vi "Read Write_Loop.vi"() -> ()   [LabVIEW 2020, in "NTV Read Write.lvlib"]
uses:
  NTV Read Write.lvlib
  Shared Code/TypeDefs/Dial_Compase heading unit circle CCW positive.ctl
  Shared Code/TypeDefs/Cluster_CMD_Direction Data.ctl
  Shared Code/TypeDefs/Cluster_Module Velocity-Direction-Rotations.ctl
  Shared Code/TypeDefs/Level_Velocity plus-minus 1.ctl
  Shared Code/TypeDefs/ENUM RB_Drive Mode IND.ctl
  Shared Code/TypeDefs/Cluster_Shooter Speed Data.ctl
  Shared Code/TypeDefs/ENUM RB_Feeder State.ctl
  Shared Code/TypeDefs/ENUM_Tube Wheel Positions.ctl
  ENUM_SEN_State.ctl
  ENUM_SEN_Action.ctl
  RoboRIO Utilities/Global_STOP.vi
  PigeonIMU/Global_SEN_Data Out.vi
  SwerveDrive/Global_CMD_ACT_Data In.vi
  Shooter/Global_CMD_ACT_Data In.vi
  Shooter/Global_ACT_Data Out.vi
  Feeder/Global_ACT_Data Out.vi
  Tube Wheel/Global_ACT_Data Out.vi
  Global_SEN_Data Out.vi
  PigeonIMU/PigeonIMU_SEN_ts.lvlib
  SwerveDrive/SwerveDrive_ACT_ts.lvlib
  Shooter/Shooter_ACT.lvlib
  Feeder/Feeder_ACT.lvlib
  Tube Wheel/Tube Wheel_ACT.lvlib
panel:
  out "Current Position":T1
  out "Feeder State":T2
  out "output cluster":T3
  out "Drive Mode":T4
  out "Run Stop":bool
  out "Direction":T5 {"Rotate(Yaw) CCW 1 CW -1" scale=1.0..-1.0; "Traverse"."Angle" scale format="%.3f"; "Traverse"."Velocity" scale=-1.0..1.0 scale format="%.1f"}
  out "Yaw":T8 scale format="%.3f"
  out "Cycle Time (S)":dbl format="%.3g"
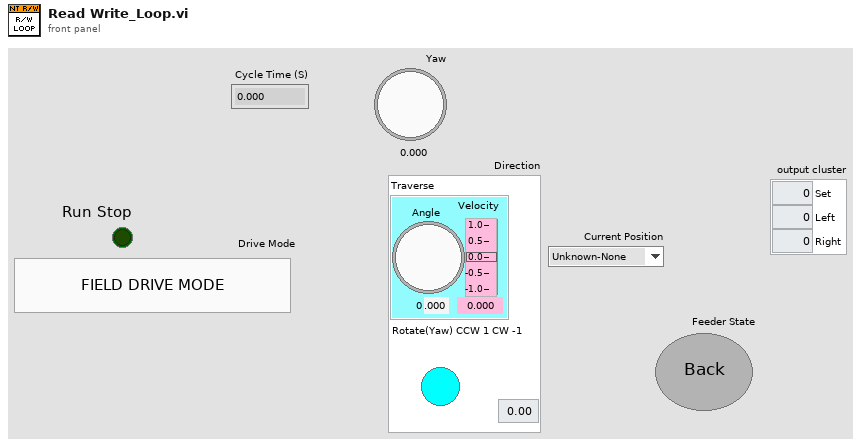
[diagram p1: front panel]
types:
  T1 = typedef "ENUM_Tube Wheel Positions.ctl" = enum16{"Unknown-None", "Tube Red A", "Tube Black B", "Tube Red C", "Tube Black D", "Tube Red E", "Tube Black F", "Load A-B", "Load B-C", "Load C-D", "Load D-E", "Load E-F", "Load F-A"}
  T2 = typedef "ENUM RB_Feeder State.ctl" = enum32{"Back", "Reversing", "Shooting"}
  T3 = typedef "Cluster_Shooter Speed Data.ctl" = cluster{"Set":dbl, "Left":dbl, "Right":dbl}
  T4 = typedef "ENUM RB_Drive Mode IND.ctl" = enum32{"Field Drive Mode", "Robot Drive Mode", "Turrent Drive Mode"}
  T5 = typedef "Cluster_CMD_Direction Data.ctl" = cluster{"Traverse":T6, "Rotate(Yaw) CCW 1 CW -1":dbl}
  T6 = typedef "Cluster_Module Velocity-Direction-Rotations.ctl" = cluster{"Velocity":T7, "Angle":T8, "Rotations Count":dbl}
  T7 = typedef "Level_Velocity plus-minus 1.ctl" = dbl
  T8 = typedef "Dial_Compase heading unit circle CCW positive.ctl" = dbl
  T9 = typedef "NTV Read Write.lvlib/ENUM_SEN_State.ctl" = enum16{"Startup", "Exchanging Variables", "Shutdown"}
  T10 = typedef "NTV Read Write.lvlib/ENUM_SEN_Action.ctl" = enum16{"No Action", "Reset Time", "Read NT Variables", "Write NT Variables"}
  T11 = cluster{"State":T9, "Previous State":T9, "Current Time":timestamp, "Previous Time":timestamp, "Start Time":timestamp, "Target Time (ms)":u32, "Cycle Time(S)":dbl, "SEN Output DBL":dbl, "Read Enable":bool}
  T12 = typedef "SwerveDrive_ACT_ts.lvlib/Cluster_CMD_ACT_Data.ctl" = cluster{"Mode":T13, "Direction":T5, "Orientation Robot(t) Field(f)":bool, "Max Translation Speed (ft/sec)":dbl, "Rotation Reduction 1-0":dbl, "Rotation Center from Robot Center":T14, "Auto Angle":T8, "Auto Target (ft)":dbl}
  T13 = typedef "ENUM_CMD_Mode Select.ctl" = enum16{"Stop", "Move", "Turret Manual"}
  T14 = typedef "Cluster_X-Y.ctl" = cluster{"X":dbl, "Y":dbl}
  T15 = typedef "Cluster_Unity Yaw-Pitch-Roll.ctl" = cluster{"Yaw":T8, "Pitch":T8, "Roll":T8}
  T16 = typedef "Feeder_ACT.lvlib/ENUM_ACT_State.ctl" = enum16{"Startup", "Back Waiting", "Push Feeding", "Retracting", "Shutdown"}
  T17 = typedef "Shooter_ACT.lvlib/Cluster_CMD_ACT_Data.ctl" = cluster{"Mode":T18, "Speed Value":dbl}
  T18 = typedef "Shooter_ACT.lvlib/ENUM_Shooter_Mode.ctl" = enum16{"Stop", "Speed Percent", "Speed RPM"}
  T19 = typedef "Shooter_ACT.lvlib/Cluster_Shooter Status.ctl" = cluster{"Left":T20, "Right":T20}
  T20 = typedef "Cluster_Speed Sensor Values.ctl" = cluster{"Velocity":T21, "Voltage":T22}
  T21 = typedef "Shooter_ACT.lvlib/Cluster_Velocity Values.ctl" = cluster{"Sensed":dbl, "Target":dbl, "Error":dbl}
  T22 = typedef "Shooter_ACT.lvlib/Cluster_Voltage Values.ctl" = cluster{"Percent":dbl, "Bus":dbl}
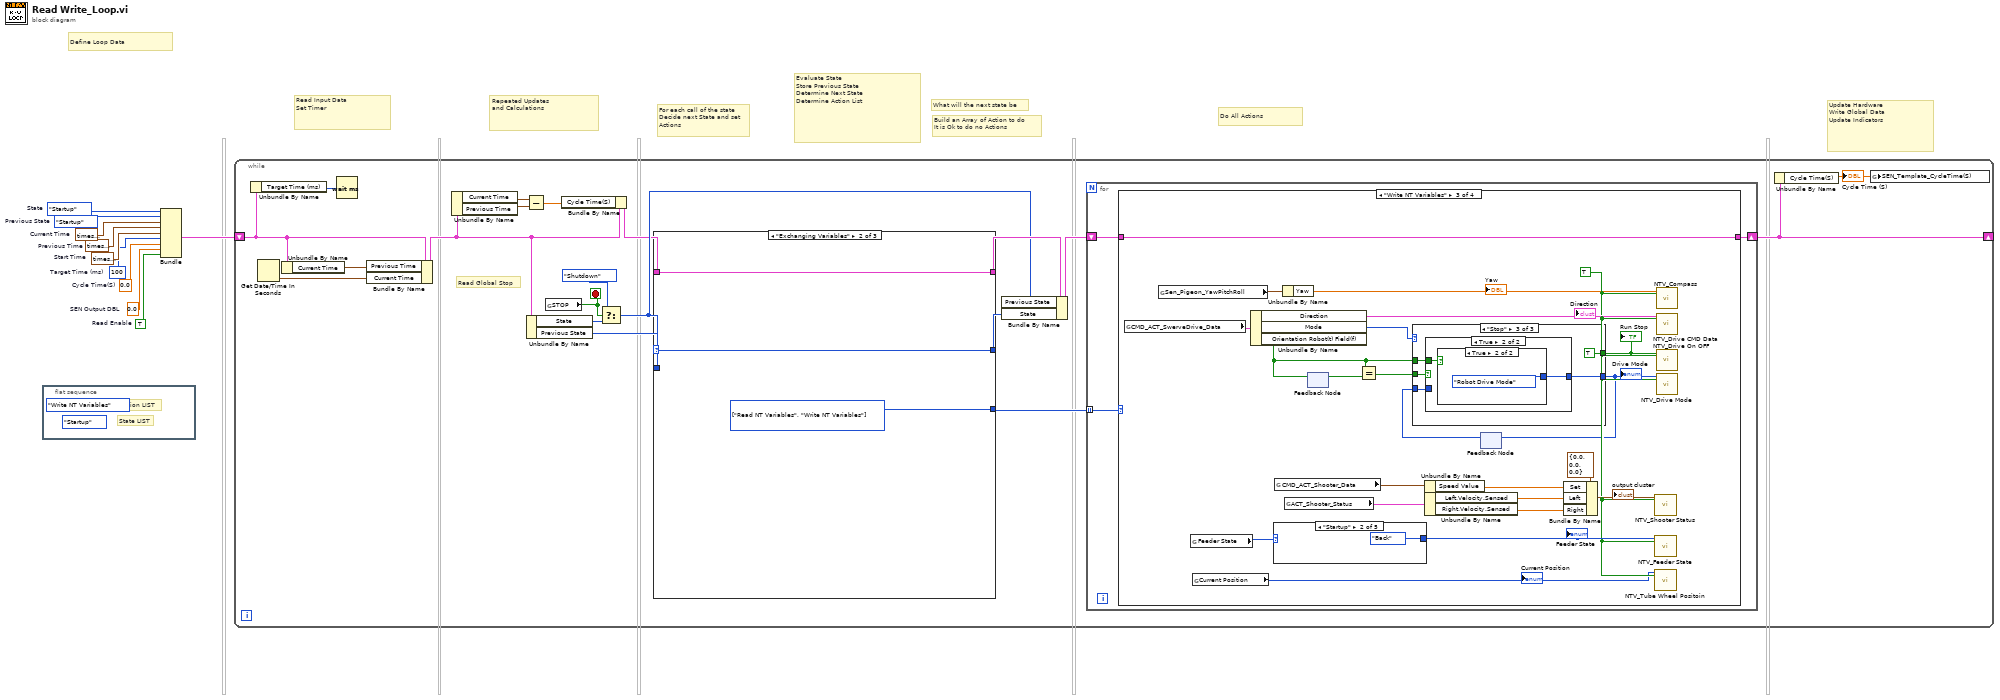
[diagram p0: block diagram]
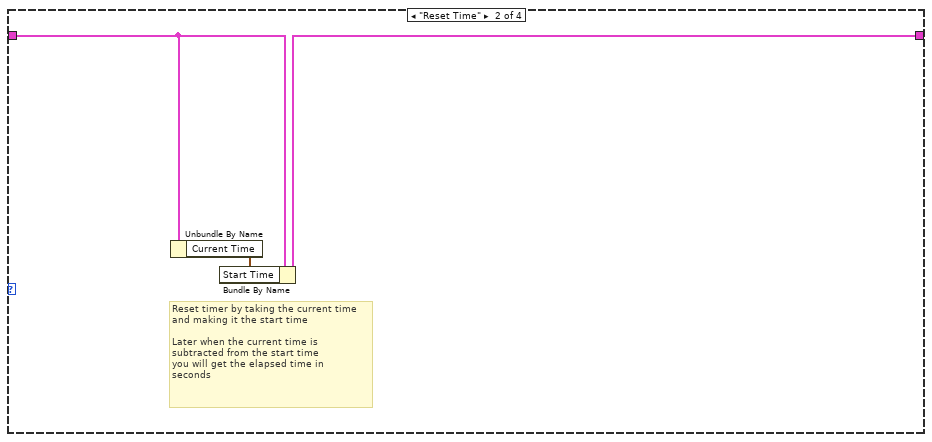
[diagram p3: hidden frame]
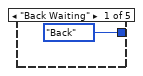
[diagram p4: hidden frame]
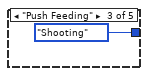
[diagram p5: hidden frame]
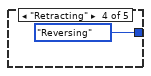
[diagram p6: hidden frame]
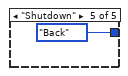
[diagram p7: hidden frame]
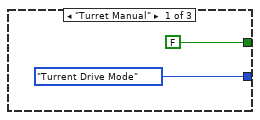
[diagram p8: hidden frame]
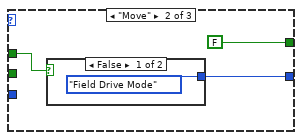
[diagram p9: hidden frame]
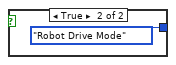
[diagram p10: hidden frame]
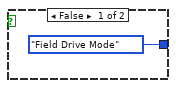
[diagram p12: hidden frame]
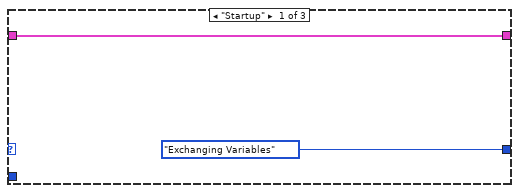
[diagram p14: hidden frame]
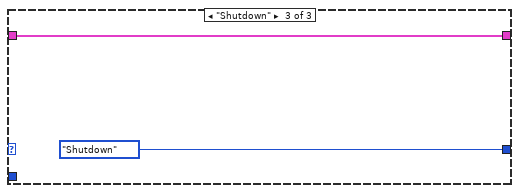
[diagram p15: hidden frame]
diagram:
  w2 = TRUE  # Read Enable
  w3 = 0.0  # Cycle Time(S)
  w4 = ENUM_SEN_State."Startup"  # Previous State
  w5 = timestamp(0 s since 1904-01-01)  # Previous Time
  w6 = u32 100  # Target Time (ms)
  w7 = 0.0  # SEN Output DBL
  w8 = timestamp(0 s since 1904-01-01)  # Start Time
  w9 = timestamp(0 s since 1904-01-01)  # Current Time
  w10 = ENUM_SEN_State."Startup"  # State
  # "Build an Array of Action to do\nIt is Ok to do no Actions"
  # "What will the next state be"
  # "For each call of the state\nDecide next State and set\nActions"
  # "Define Loop Data"
  # "Repeated Updates\nand Calculations"
  # "Read Input Data\nSet Timer"
  # "Evaluate State\nStore Previous State\nDetermine Next State\nDetermine Action List"
  # "Do All Actions"
  # "Update Hardware\nWrite Global Data\nUpdate Indicators"
  n1 = flat-sequence {
    frame #0 {
      (unwired) ENUM_SEN_State."Startup" ("State")
      (unwired) ENUM_SEN_Action."Write NT Variables" ("Action")
      # "State LIST"
      # "Action LIST"
    }
  }
  n2 = Bundle("State"=w10, "Previous State"=w4, "Current Time"=w9, "Previous Time"=w5, "Start Time"=w8, "Target Time (ms)"=w6, "Cycle Time(S)"=w3, "SEN Output DBL"=w7, "Read Enable"=w2) -> (w1:T11)  [unwired: 1 in]
  n3 = while {
    shift-right: [w11] -> _
    shift-left: w1 -> [w21]
    stop <- w26 stop-if-true
    # "Read Global Stop"
    n4 = Unbundle By Name(w21) -> ("Target Time (ms)"=w23:u32)
    n5 = Get Date/Time In Seconds() -> (seconds since 1Jan1904=w30:timestamp)
    n6 = Unbundle By Name(w21) -> ("Current Time"=w22:timestamp)
    n7 = Wait (ms)(milliseconds to wait=w23) -> ()  [unwired: 1 out]
    n8 = Bundle By Name(cluster=w21, "Previous Time"=w22, "Current Time"=w30) -> (w16:T11)
    n9 = Unbundle By Name(w16) -> ("Current Time"=w17:timestamp, "Previous Time"=w18:timestamp)
    n10 = Subtract(x=w17, y=w18) -> (x-y=w14:dbl)
    n11 = Unbundle By Name(w16) -> ("State"=w24:T9, "Previous State"=w20:T9)
    n12 = global read "Global_STOP.vi" "STOP"() -> (w26:bool)
    n13 = Bundle By Name(cluster=w16, "Cycle Time(S)"=w14) -> (w15:T11)
    n14 = Select(t=ENUM_SEN_State."Shutdown" ("State"), s=w26, f=w24) -> (s? t:f=w19:T9)
    n15 = case shown="\"Exchanging Variables\"" w19 {
      selector: w19 -> [_ w86 _]
      tunnel: w15 -> [w85 w88 w90]
      tunnel: [w85 w88 w90] -> w28
      tunnel: [ENUM_SEN_State."Exchanging Variables" ("State") w86 ENUM_SEN_State."Shutdown" ("State")] -> w27
      tunnel: [_ w87 _] -> w13
      tunnel: w20 -> [_ _ _]
      frame "Startup" {
      }
      frame "Exchanging Variables" {
        w87 = T10[] [enum."Read NT Variables", enum."Write NT Variables"] items=["No Action", "Reset Time", "Read NT Variables", "Write NT Variables"] ("Actions")
      }
      frame "Shutdown" {
      }
    }
    n16 = Bundle By Name(cluster=w28, "Previous State"=w19, "State"=w27) -> (w29:T11)
    n17 = for {
      tunnel: w13 -> [w33] mode=indexing
      shift-right: [w32] -> w11
      shift-left: w29 -> [w31]
      n18 = case shown="\"Write NT Variables\"" w33 {
        tunnel: w31 -> [w34 w37 w60 w83]
        tunnel: [w34 w36 w60 w83] -> w32
        frame "No Action" {
        }
        frame "Reset Time" {
          # "Reset timer by taking the current time\nand making it the start time\n\nLater when the current time is \nsubtracted from the start time\nyou will get the elapsed time in \nseconds"
          n19 = Unbundle By Name(w37) -> ("Current Time"=w35:timestamp)
          n20 = Bundle By Name(cluster=w37, "Start Time"=w35) -> (w36:T11)
        }
        frame "Write NT Variables" {
          w44 = TRUE ("Read(f) Write(t)")
          n21 = global read "Global_CMD_ACT_Data In.vi" "CMD_ACT_SwerveDrive_Data"() -> (w57:T12)
          n22 = global read "Global_SEN_Data Out.vi" "Sen_Pigeon_YawPitchRoll"() -> (w59:T15)
          n23 = global read "Global_ACT_Data Out.vi" "Feeder State"() -> (w47:T16)
          n24 = global read "Global_ACT_Data Out.vi" "Current Position"() -> (w43:T1)
          "Current Position" <- w43
          n25 = Unbundle By Name(w57) -> ("Direction"=w56:T5, "Mode"=w55:T13, "Orientation Robot(t) Field(f)"=w39:bool)
          "Direction" <- w56
          n26 = case shown="\"Startup\"" w47 {
            tunnel: [ENUM_RB_Feeder_State."Back" ("Feeder State") ENUM_RB_Feeder_State."Back" ("Feeder State") ENUM_RB_Feeder_State."Shooting" ("Feeder State") ENUM_RB_Feeder_State."Reversing" ("Feeder State") ENUM_RB_Feeder_State."Back" ("Feeder State")] -> w46
            frame "Back Waiting" {
            }
            frame "Startup" {
            }
            frame "Push Feeding" {
            }
            frame "Retracting" {
            }
            frame "Shutdown" {
            }
          }
          "Feeder State" <- w46
          n27 = global read "Global_CMD_ACT_Data In.vi" "CMD_ACT_Shooter_Data"() -> (w54:T17)
          n28 = Unbundle By Name(w59) -> ("Yaw"=w58:T8)
          "Yaw" <- w58
          n29 = global read "Global_ACT_Data Out.vi" "ACT_Shooter_Status"() -> (w53:T19)
          n30 = feedback-in #1(w39) -> ()
          n31 = feedback #1() -> (w40:bool)  [unwired: 1 in]
          n32 = Equal?(x=w39, y=w40) -> (x = y?=w38:bool)
          n33 = Unbundle By Name(w54) -> ("Speed Value"=w50:dbl)
          n34 = Unbundle By Name(w53) -> ("Left.Velocity.Sensed"=w49:dbl, "Right.Velocity.Sensed"=w48:dbl)
          n35 = feedback #2() -> (w41:T4)  [unwired: 1 in]
          n36 = case shown="\"Stop\"" w55 {
            tunnel: w39 -> [_ w70 w77]
            tunnel: [ENUM_RB_Drive_Mode_IND."Turrent Drive Mode" ("Drive Mode") w69 w76] -> w42
            tunnel: [FALSE ("Run Stop") FALSE ("Run Stop") TRUE ("Run Stop")] -> w45
            tunnel: w41 -> [_ _ w73]
            tunnel: w38 -> [_ _ w74]
            frame "Turret Manual" {
            }
            frame "Move" {
              n37 = case shown="False" w70 {
                tunnel: [ENUM_RB_Drive_Mode_IND."Field Drive Mode" ("Drive Mode") ENUM_RB_Drive_Mode_IND."Robot Drive Mode" ("Drive Mode")] -> w69
                frame False {
                }
                frame True {
                }
              }
            }
            frame "Stop" {
              n38 = case shown="True" w74 {
                tunnel: w77 -> [_ w80]
                tunnel: [w78 w79] -> w76
                tunnel: w73 -> [w78 _]
                frame False {
                }
                frame True {
                  n39 = case shown="True" w80 {
                    tunnel: [ENUM_RB_Drive_Mode_IND."Field Drive Mode" ("Drive Mode") ENUM_RB_Drive_Mode_IND."Robot Drive Mode" ("Drive Mode")] -> w79
                    frame False {
                    }
                    frame True {
                    }
                  }
                }
              }
            }
          }
          "Run Stop" <- w45
          "Drive Mode" <- w42
          n40 = feedback-in #2(w42) -> ()
          n41 = Bundle By Name(cluster=T3 {"Set"=0.0, "Left"=0.0, "Right"=0.0} ("Shooter Speed"), "Set"=w50, "Left"=w49, "Right"=w48) -> (w51:T3)
          "output cluster" <- w51
          n42 = call "NTV_Shooter Status.vi"("Read(f) Write(t)"=w44, "Shooter Speed"=w51) -> ()  [unwired: 9 in, 1 out]
          n43 = call "NTV_Feeder State.vi"("Read(f) Write(t)"=w44, "Feeder State"=w46) -> ()  [unwired: 9 in, 1 out]
          n44 = call "NTV_Tube Wheel Positoin.vi"("Read(f) Write(t)"=w44, "Tube Wheel Positions"=w43) -> ()  [unwired: 9 in, 1 out]
          n45 = call "NTV_Compass.vi"("Read(f) Write(t)"=w44, "Compass"=w58) -> ()  [unwired: 9 in, 1 out]
          n46 = call "NTV_Drive CMD Data.vi"("Read(f) Write(t)"=w44, "Comand Data"=w56) -> ()  [unwired: 9 in, 1 out]
          n47 = call "NTV_Drive On OFF.vi"("Read(f) Write(t)"=w44, "Run Stop"=w45) -> ()  [unwired: 9 in, 1 out]
          n48 = call "NTV_Drive Mode.vi"("Read(f) Write(t)"=w44, "Drive Mode"=w42) -> ()  [unwired: 9 in, 1 out]
        }
        frame "Read NT Variables" {
        }
      }
    }
    n49 = Unbundle By Name(w11) -> ("Cycle Time(S)"=w12:dbl)
    "Cycle Time (S)" <- w12
    n50 = global write "Global_SEN_Data Out.vi" "SEN_Template_CycleTime(S)"(w12) -> ()
  }
